vi "Bin Size Dialog.vi"(0 "Enable":bool=TRUE, 5 "error in (no error)":errorcluster) -> (17 "Bin Size":dbl format="%#g", 18 "OK":bool, 19 "error out":errorcluster)   [LabVIEW 2019]
doc: "Displays a standard dialog box that prompts users to enter information, such as a user name and password.\n--------------------\n\nThis Express VI is configured as follows:\n\nMessage to Display to the User:Enter new histogram bin size:\nThe inputs are: \nNumber: Bin Size"
panel:
  in  "Bin Size":dbl format="%#g"
  out "String":string="Enter new histogram bin size:"
  in  "Cancel":bool
  in  "OK2":bool
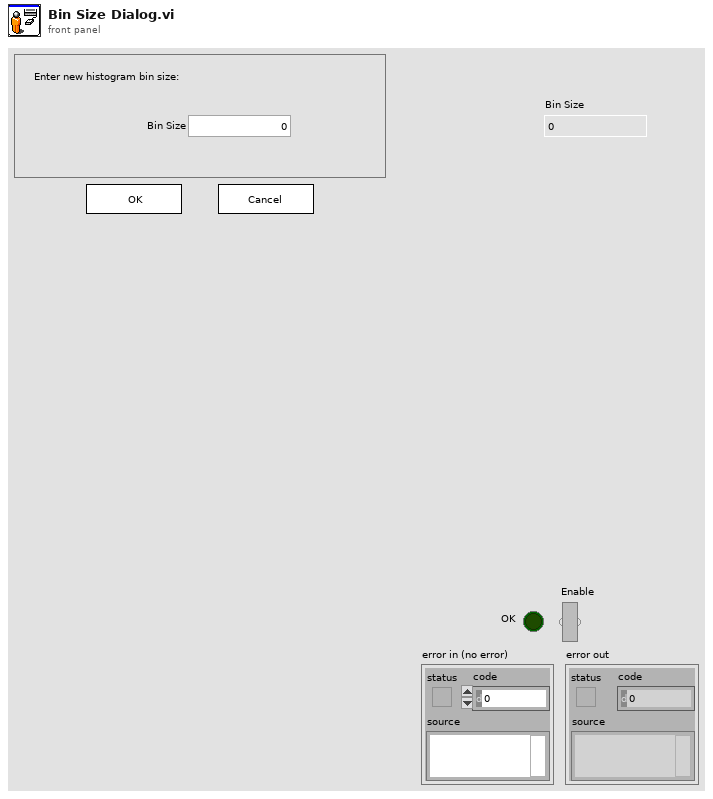
[diagram p1: front panel]
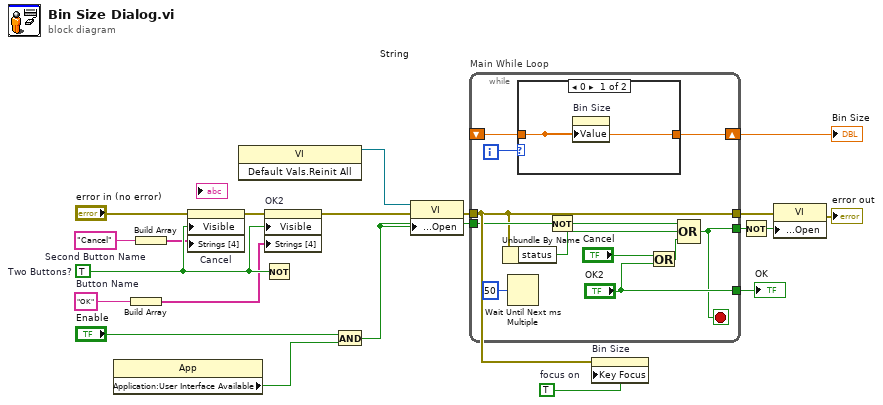
[diagram p0: block diagram]
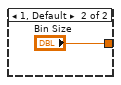
[diagram p2: hidden frame]
diagram:
  w2 = TRUE  # focus on
  w14 = "Cancel"  # Second Button Name
  w12 = "OK"  # Button Name
  w20 = TRUE  # Two Buttons?
  n1 = property class="App"() -> ("Application:User Interface Available"=w5:bool)  [unwired: 2 in, 2 out]
  n2 = Build Array(w12) -> (w13:string[])
  n3 = Build Array(w14) -> (w15:string[])
  n4 = property on="Cancel" class="Bool"(error in="error in (no error)", "Visible"=w20, "Strings [4]"=w15) -> (error out=w18:errorcluster)  [unwired: 1 in, 1 out]
  n5 = invoke class="VI" method="Default Vals.Reinit All"() -> (reference out=w4:refnum<vi>)  [unwired: 3 in, 2 out]
  n6 = Not(x=w20) -> ()  [unwired: 1 out]
  n7 = property on="OK2" class="Bool"(error in=w18, "Visible"=w20, "Strings [4]"=w13) -> (error out=w1:errorcluster)  [unwired: 1 in, 1 out]
  n8 = And(x="Enable", y=w5) -> (x .and. y?=w6:bool)
  n9 = property class="VI"(reference=w4, error in=w1, "Front Panel Window:Open"=w6) -> (error out=w11:errorcluster)  [unwired: 1 out]
  n10 = while "Main While Loop" {
    tunnel: ["OK2"] -> w19
    tunnel: w6 -> [w29]
    tunnel: [w27] -> w16
    tunnel: w11 -> [w26]
    tunnel: [w26] -> w9
    shift-right: [w23] -> w3
    shift-left: _ -> [w21]
    i -> [w22]
    stop <- w27 stop-if-true
    n11 = Unbundle By Name(w26) -> ("status"=w24:bool)
    n12 = Wait Until Next ms Multiple(millisecond multiple=u32 50) -> ()  [unwired: 1 out]
    n13 = case shown="0" w22 {
      tunnel: [w33 "Bin Size"] -> w23
      tunnel: w21 -> [w33 _]
      frame 0 {
        n14 = property on="Bin Size" class="DigNum (strict)"("Value"=w33) -> ()  [unwired: 2 in, 2 out]
      }
      frame 1, Default {
      }
    }
    n15 = Not(x=w29) -> (.not. x?=w28:bool)
    n16 = Or(x="Cancel", y="OK2") -> (x .or. y?=w25:bool)
    n17 = Compound Arithmetic op=OR(w28, w24, w25) -> (w27:bool)
  }
  "OK" <- w19
  "Bin Size" <- w3
  n18 = property on="Bin Size" class="DigNum (strict)"(error in=w11, "Key Focus"=w2) -> ()  [unwired: 1 in, 2 out]
  n19 = Not(x=w16) -> (.not. x?=w17:bool)
  n20 = property class="VI"(error in=w9, "Front Panel Window:Open"=w17) -> (error out=→"error out":errorcluster)  [unwired: 1 in, 1 out]
